vi "checksum(SubVI).vi"(11 "response":string) -> (3 "CHKSUM":string)   [LabVIEW 2018]
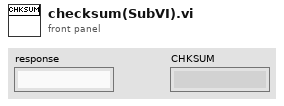
[diagram p1: front panel]
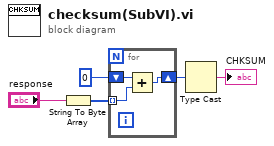
[diagram p0: block diagram]
diagram:
  n1 = String To Byte Array(string="response") -> (unsigned byte array=w3:u8[])
  n2 = for {
    tunnel: w3 -> [w6] mode=indexing
    shift-right: [w8] -> w5
    shift-left: u8 0 -> [w7]
    n3 = Add(x=w7, y=w6) -> (x+y=w8:u8)
  }
  n4 = Type Cast(x=w5) -> (*(type *) &x=→"CHKSUM":string)  [unwired: 1 in]
